vi "Heart Rate Monitor.vi"() -> ()   [LabVIEW 2012]
doc: "The Heart Rate Monitor application that is composed of three major sections: <b>Data Acquisition</b>, <b>Data Processing</b>, and <b>Data Presentation</b>."
uses:
  Controls/Detect Threshold Control.ctl
panel:
  out "Data":dynamicdata(graph) caption="Heart Rate Monitor"
  out "BPM":string="Calibrating..."
  in  "Simulate Heart Beat?":bool caption="Simulate?"
  in  "Stop":bool
  out "Pulse":bool
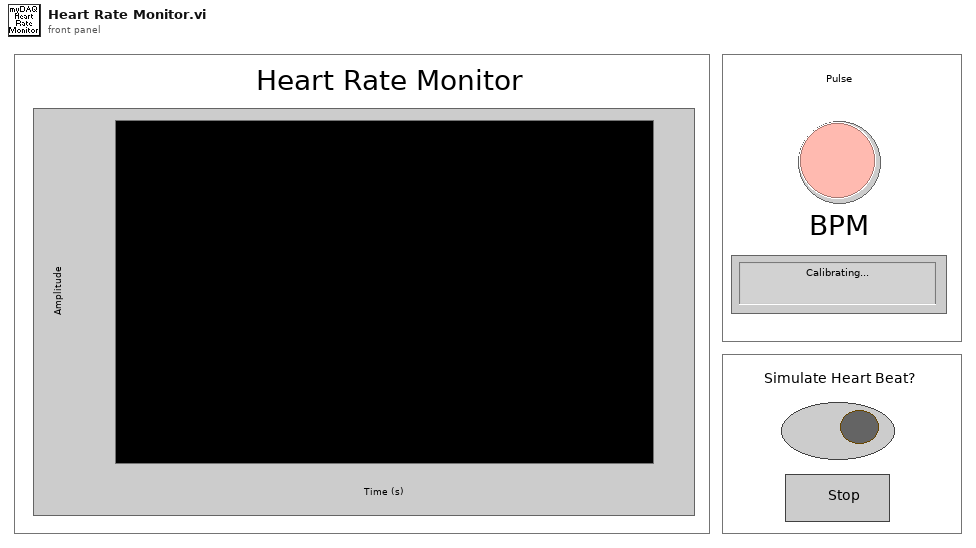
[diagram p1: front panel]
types:
  T1 = typedef "Detect Threshold Control.ctl" = enum16{"Get Threshold", "Pulse Found", "Pulse Not Found"}
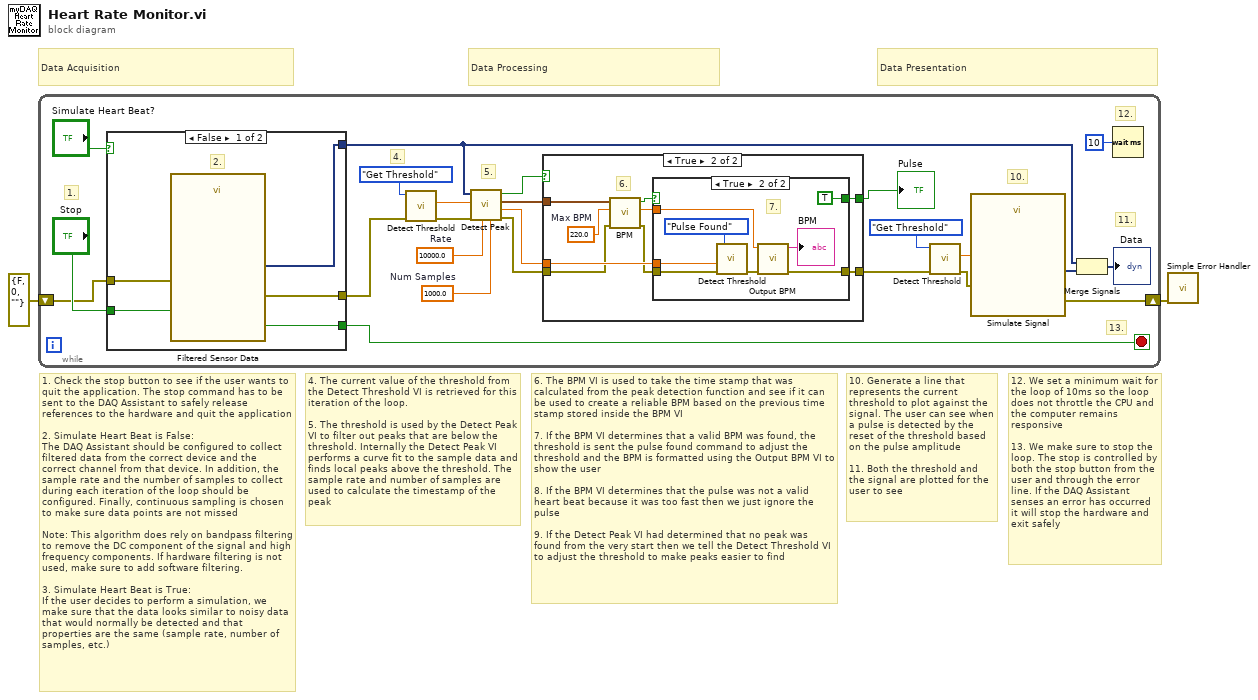
[diagram p0: block diagram]
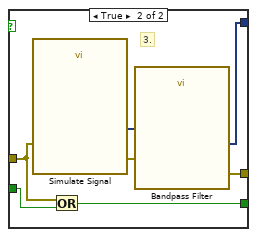
[diagram p2: hidden frame]
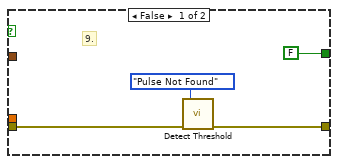
[diagram p3: hidden frame]
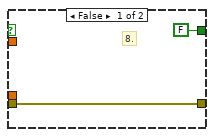
[diagram p4: hidden frame]
diagram:
  # "Data Presentation"
  # "Data Processing"
  # "Data Acquisition"
  # "12. We set a minimum wait for the loop of 10ms so the loop does not throttle the CPU and the computer remains responsive\n\n13. We make sure to stop the loop. The stop is controlled by both the stop button from the user and through the error line. If the DAQ Assistant senses an error has occurred it will stop the hardware and exit safely"
  # "10. Generate a line that represents the current threshold to plot against the signal. The user can see when a pulse is detected by the reset of the threshold based on the pulse amplitude\n\n11. Both the threshold and the signal are plotted for the user to see"
  # "6. The BPM VI is used to take the time stamp that was calculated from the peak detection function and see if it can be used to create a reliable BPM based on the previous time stamp stored inside the BPM VI \n\n7. If the BPM VI determines that a valid BPM was found, the threshold is sent the pulse found command to adjust the threshold and the BPM is formatted using the Output BPM VI to show the user\n\n8. If the BPM VI determines that the pulse was not a valid heart beat because it was too fast then we just ignore the pulse\n\n9. If the Detect Peak VI had determined that no peak was found from the very start then we tell the Detect Threshold VI to adjust the threshold to make peaks easier to find"
  # "4. The current value of the threshold from the Detect Threshold VI is retrieved for this iteration of the loop.\n\n5. The threshold is used by the Detect Peak VI to filter out peaks that are below the threshold. Internally the Detect Peak VI performs a curve fit to the sample data and finds local peaks above the threshold. The sample rate and number of samples are used to calculate the timestamp of the peak"
  # "1. Check the stop button to see if the user wants to quit the application. The stop command has to be sent to the DAQ Assistant to safely release references to the hardware and quit the application\n\n2. Simulate Heart Beat is False:\nThe DAQ Assistant should be configured to collect filtered data from the correct device and the correct channel from that device. In addition, the sample rate and the number of samples to collect during each iteration of the loop should be configured. Finally, continuous sampling is chosen to make sure data points are not missed\n\nNote: This algorithm does rely on bandpass filtering to remove the DC component of the signal and high frequency components. If hardware filtering is not used, make sure to add software filtering.\n\n3. Simulate Heart Beat is True:\nIf the user decides to perform a simulation, we make sure that the data looks similar to noisy data that would normally be detected and that properties are the same (sample rate, number of samples, etc.)"
  n1 = while {
    shift-right: [w4] -> w2
    shift-left: errorcluster {"status"=FALSE, "code"=0, "source"=""} ("error out") -> [w13]
    stop <- w3 stop-if-true
    w14 = 1000.0  # Num Samples
    w15 = 10000.0  # Rate
    # "5."
    # "13."
    # "12."
    # "11."
    # "10."
    # "4."
    # "1."
    n2 = case shown="False" "Simulate Heart Beat?" {
      tunnel: [w31 w32] -> w3
      tunnel: "Stop" -> [w30 w34]
      tunnel: [w28 w38] -> w8
      tunnel: [w27 w35] -> w9
      tunnel: w13 -> [w29 w33]
      frame False {
        # "2."
        n3 = call "Filtered Sensor Data"("error in"=w29, "stop (F)"=w30) -> ("data"=w28:dynamicdata, "stopped"=w31:bool, "error out"=w27:errorcluster)  [unwired: 14 in, 1 out]
      }
      frame True {
        # "3."
        n4 = call "Simulate Signal"("error in (no error)"=w33) -> ("Simulated Sensor"=w37:dynamicdata, "error out"=w36:errorcluster)  [unwired: 13 in]
        n5 = Or(x=w33, y=w34) -> (x .or. y?=w32:bool)
        n6 = call "Bandpass Filter"("error in (no error)"=w36, "Signal"=w37) -> ("error out"=w35:errorcluster, "Filtered Signal"=w38:dynamicdata)  [unwired: 8 in]
      }
    }
    n7 = call "Detect Threshold.vi"("error in (no error)"=w9, "Action"=Detect_Threshold_Control."Get Threshold") -> ("error out"=w17:errorcluster, "Threshold"=w18:dbl)  [unwired: 4 in]
    n8 = call "Detect Peak.vi"("Num Samples"=w14, "Rate"=w15, "error in (no error)"=w17, "Threshold"=w18, "Filtered Signal"=w8) -> ("error out"=w16:errorcluster, "Peak Amplitude"=w22:dbl, "Peak Time Stamp"=w23:timestamp, "Peak Found?"=w12:bool)  [unwired: 3 in]
    n9 = case shown="True" w12 {
      tunnel: w23 -> [_ w51]
      tunnel: w22 -> [_ w49]
      tunnel: w16 -> [w41 w43]
      tunnel: [w40 w46] -> w7
      tunnel: [FALSE w44] -> w10
      frame False {
        # "9."
        n10 = call "Detect Threshold.vi"("error in (no error)"=w41, "Action"=Detect_Threshold_Control."Pulse Not Found") -> ("error out"=w40:errorcluster)  [unwired: 4 in, 1 out]
      }
      frame True {
        w50 = 220.0  # Max BPM
        # "6."
        n11 = call "BPM.vi"("error in (no error)"=w43, "Max BPM Threshold"=w50, "Time Stamp"=w51) -> ("error out"=w45:errorcluster, "BPM"=w47:dbl, "Below MAX BPM Threshold?"=w48:bool)  [unwired: 2 in]
        n12 = case shown="True" w48 {
          tunnel: w49 -> [_ w61]
          tunnel: w47 -> [_ w55]
          tunnel: [w53 w58] -> w46
          tunnel: w45 -> [w53 w57]
          tunnel: [FALSE TRUE] -> w44
          frame False {
            # "8."
          }
          frame True {
            # "7."
            n13 = call "Detect Threshold.vi"("error in (no error)"=w57, "Amplitude"=w61, "Action"=Detect_Threshold_Control."Pulse Found") -> ("error out"=w59:errorcluster)  [unwired: 3 in, 1 out]
            n14 = call "Output BPM.vi"("error in (no error)"=w59, "BPM (input)"=w55) -> ("error out"=w58:errorcluster, "BPM (output)"=→"BPM":string)  [unwired: 4 in]
          }
        }
      }
    }
    "Pulse" <- w10
    n15 = call "Detect Threshold.vi"("error in (no error)"=w7, "Action"=Detect_Threshold_Control."Get Threshold") -> ("error out"=w6:errorcluster, "Threshold"=w19:dbl)  [unwired: 4 in]
    n16 = call "Simulate Signal"("Offset"=w19, "error in (no error)"=w6) -> ("Peak Threshold"=w11:dynamicdata, "error out"=w4:errorcluster)  [unwired: 12 in]
    n17 = Merge Signals(w8, w11) -> (→"Data":dynamicdata)
    n18 = Wait (ms)(milliseconds to wait=u32 10) -> ()  [unwired: 1 out]
  }
  n19 = call <vilib>:"Simple Error Handler.vi"("error in (no error)"=w2) -> ()  [unwired: 4 in, 5 out]
